vi "Autonomous Independent.vi"   [LabVIEW 2017] (continued)
                tunnel: [w1142] -> w956
                tunnel: [w1141] -> w955
                tunnel: w958 -> [w1156]
                tunnel: w957 -> [w1155]
                tunnel: [w1154] -> w954
                tunnel: [w1153] -> w953
                tunnel: [w1152] -> w952
                tunnel: w956 -> [w1152]
                tunnel: [w1151] -> w951
                tunnel: w955 -> [w1151]
                tunnel: w954 -> [w1164]
                tunnel: w953 -> [w1163]
                tunnel: [w1162] -> w950
                tunnel: w952 -> [w1162]
                tunnel: [w1161] -> w949
                tunnel: w951 -> [w1161]
                tunnel: [w1160] -> w948
                tunnel: [w1159] -> w947
                tunnel: w950 -> [w1184]
                tunnel: w949 -> [w1183]
                tunnel: [w1182] -> w946
                tunnel: w948 -> [w1182]
                tunnel: [w1181] -> w945
                tunnel: w947 -> [w1181]
                tunnel: [w1180] -> w944
                tunnel: [w1179] -> w943
                tunnel: w946 -> [w1192]
                tunnel: w945 -> [w1191]
                tunnel: w944 -> [w1190]
                tunnel: w943 -> [w1189]
                tunnel: [w1188] -> w942
                tunnel: [w1187] -> w941
                tunnel: [w1186] -> w940
                tunnel: [w1185] -> w939
                tunnel: [w1198] -> w935
                tunnel: w942 -> [w1198]
                tunnel: [w1197] -> w936
                tunnel: w941 -> [w1197]
                tunnel: [w1196] -> w937
                tunnel: w940 -> [w1196]
                tunnel: [w1195] -> w938
                tunnel: w939 -> [w1195]
                tunnel: [w1206] -> w934
                tunnel: [w1202] -> w933
                tunnel: [w1201] -> w932
                tunnel: [w1205] -> w931
                tunnel: w938 -> [w1201]
                tunnel: w937 -> [w1202]
                tunnel: w936 -> [w1203]
                tunnel: w935 -> [w1204]
                tunnel: w934 -> [w1214]
                tunnel: w933 -> [w1213]
                tunnel: w932 -> [w1212]
                tunnel: [w1211] -> w930
                tunnel: w931 -> [w1211]
                tunnel: [w1210] -> w929
                tunnel: [w1209] -> w928
                tunnel: [w1208] -> w927
                tunnel: w930 -> [w1224]
                tunnel: w929 -> [w1223]
                tunnel: w928 -> [w1222]
                tunnel: w927 -> [w1221]
                tunnel: [w1220] -> w926
                tunnel: [w1219] -> w925
                tunnel: [w1218] -> w924
                tunnel: [w1217] -> w923
                tunnel: w926 -> [w1233]
                tunnel: w925 -> [w1232]
                tunnel: [w1231] -> w922
                tunnel: w924 -> [w1231]
                tunnel: [w1230] -> w921
                tunnel: w923 -> [w1230]
                tunnel: [w1229] -> w920
                tunnel: [w1228] -> w919
                tunnel: w922 -> [w1246]
                tunnel: w921 -> [w1245]
                tunnel: [w1244] -> w918
                tunnel: w920 -> [w1244]
                tunnel: [w1243] -> w917
                tunnel: w919 -> [w1243]
                tunnel: [w1242] -> w916
                tunnel: [w1241] -> w915
                tunnel: w918 -> [w1260]
                tunnel: w917 -> [w1259]
                tunnel: w916 -> [w1258]
                tunnel: w915 -> [w1257]
                tunnel: [w1256] -> w914
                tunnel: [w1255] -> w913
                tunnel: [w1254] -> w912
                tunnel: [w1253] -> w911
                tunnel: [w1266] -> w910
                tunnel: w914 -> [w1267]
                tunnel: [w1265] -> w909
                tunnel: w913 -> [w1265]
                tunnel: [w1264] -> w908
                tunnel: w912 -> [w1264]
                tunnel: [w1263] -> w907
                tunnel: w911 -> [w1263]
                tunnel: [w1278] -> w906
                tunnel: w910 -> [w1278]
                tunnel: [w1277] -> w905
                tunnel: w909 -> [w1277]
                tunnel: [w1276] -> w904
                tunnel: w908 -> [w1276]
                tunnel: [w1275] -> w903
                tunnel: w907 -> [w1275]
                tunnel: w906 -> [w1284]
                tunnel: w905 -> [w1283]
                tunnel: w904 -> [w1282]
                tunnel: w903 -> [w1281]
                frame #0 {
                  n287 = call "PID Distance.vi"("Distance"=20.0, "Angle"=0.0, "RightEncoder"=w1015, "LeftEncoder"=w1016, "GyroDevRef"=w1018, "RobotDriveDevRef"=w1017) -> ("RightEncoder 2"=w1011:T11, "LeftEncoder 2"=w1012:T11, "GyroDevRef 2"=w1013:T8, "RobotDriveDevRef 2"=w1014:T1)  [unwired: 2 in]
                }
                frame #1 {
                  w1027 = 0.0 ("Left axis value")
                  n288 = global write "Robot Global Data.vi" "Raise_Mast"(TRUE ("Current State")) -> ()
                  n289 = Wait (ms)(milliseconds to wait=u32 100) -> ()  [unwired: 1 out]
                  n290 = call <vilib>:"WPI_RobotDriveTankDrive.vi"("Right axis value"=w1027, "Left axis value"=w1027, "RobotDriveDevRef"=w1025) -> ("RobotDriveDevRef"=w1026:T1)  [unwired: 6 in, 2 out]
                }
                frame #2 {
                  n291 = call "PID turning.vi"("Angle"=-50.0, "GyroDevRef"=w1032, "RobotDriveDevRef"=w1031) -> ("GyroDevRef 2"=w1029:T8, "RobotDriveDevRef 2"=w1030:T1)  [unwired: 7 in]
                  n292 = global write "Robot Global Data.vi" "Raise_Mast"(TRUE ("Current State")) -> ()
                }
                frame #3 {
                  w1038 = 0.0 ("Left axis value")
                  n293 = call <vilib>:"WPI_EncoderReset.vi"("EncoderDevRef"=w1043) -> ("EncoderDevRef"=w1040:T11)  [unwired: 9 in, 1 out]
                  n294 = call <vilib>:"WPI_EncoderReset.vi"("EncoderDevRef"=w1042) -> ("EncoderDevRef"=w1041:T11)  [unwired: 9 in, 1 out]
                  n295 = Wait (ms)(milliseconds to wait=u32 10) -> ()  [unwired: 1 out]
                  n296 = call <vilib>:"WPI_RobotDriveTankDrive.vi"("Right axis value"=w1038, "Left axis value"=w1038, "RobotDriveDevRef"=w1044) -> ("RobotDriveDevRef"=w1039:T1)  [unwired: 6 in, 2 out]
                }
                frame #4 {
                  n297 = call "PID Distance.vi"("Distance"=75.0, "Angle"=-50.0, "RightEncoder"=w1051, "LeftEncoder"=w1050, "GyroDevRef"=w1053, "RobotDriveDevRef"=w1052) -> ("RightEncoder 2"=w1046:T11, "LeftEncoder 2"=w1047:T11, "GyroDevRef 2"=w1049:T8, "RobotDriveDevRef 2"=w1048:T1)  [unwired: 2 in]
                  n298 = global write "Robot Global Data.vi" "Raise_Mast"(TRUE ("Current State")) -> ()
                }
                frame #5 {
                  n299 = global read "Robot Global Data.vi" "Axes"() -> (w1063:dbl[])
                  n300 = global write "Robot Global Data.vi" "Raise_Mast"(TRUE ("Current State")) -> ()
                  n301 = Array To Cluster(array=w1063) -> (cluster=w1064:T15)
                  n302 = Bundle By Name(cluster=w1064, "Axes[1]"=-1.0) -> (w1061:T15)
                  n303 = Cluster To Array(cluster=w1061) -> (array=w1062:dbl[])
                  n304 = call "PID turning.vi"("Angle"=0.0, "GyroDevRef"=w1065, "RobotDriveDevRef"=w1066) -> ("GyroDevRef 2"=w1057:T8, "RobotDriveDevRef 2"=w1058:T1)  [unwired: 7 in]
                  n305 = global write "Robot Global Data.vi" "Axes"(w1062) -> ()
                }
                frame #6 {
                  n306 = global read "Robot Global Data.vi" "Axes"() -> (w1073:dbl[])
                  n307 = global write "Robot Global Data.vi" "Lift_Position"(2.0) -> ()
                  n308 = Array To Cluster(array=w1073) -> (cluster=w1072:T15)
                  n309 = Bundle By Name(cluster=w1072, "Axes[1]"=-1.0) -> (w1075:T15)
                  n310 = Cluster To Array(cluster=w1075) -> (array=w1074:dbl[])
                  n311 = call <vilib>:"WPI_EncoderReset.vi"("EncoderDevRef"=w1070) -> ("EncoderDevRef"=w1080:T11)  [unwired: 9 in, 1 out]
                  n312 = global write "Robot Global Data.vi" "Axes"(w1074) -> ()
                  n313 = call <vilib>:"WPI_EncoderReset.vi"("EncoderDevRef"=w1071) -> ("EncoderDevRef"=w1081:T11)  [unwired: 9 in, 1 out]
                }
                frame #7 {
                  n314 = call "PID Distance.vi"("Distance"=50.0, "Angle"=0.0, "RightEncoder"=w1085, "LeftEncoder"=w1086, "GyroDevRef"=w1088, "RobotDriveDevRef"=w1087) -> ("RightEncoder 2"=w1082:T11, "LeftEncoder 2"=w1083:T11, "GyroDevRef 2"=w1084:T8, "RobotDriveDevRef 2"=w1089:T1)  [unwired: 2 in]
                }
                frame #8 {
                  w1104 = 0.0 ("Left axis value")
                  n315 = global read "Robot Global Data.vi" "Axes"() -> (w1100:dbl[])
                  n316 = global write "Robot Global Data.vi" "Lift_Position"(2.0) -> ()
                  n317 = Wait (ms)(milliseconds to wait=u32 250) -> ()  [unwired: 1 out]
                  n318 = Array To Cluster(array=w1100) -> (cluster=w1099:T15)
                  n319 = Bundle By Name(cluster=w1099, "Axes[1]"=1.0) -> (w1097:T15)
                  n320 = Cluster To Array(cluster=w1097) -> (array=w1096:dbl[])
                  n321 = call <vilib>:"WPI_RobotDriveTankDrive.vi"("Right axis value"=w1104, "Left axis value"=w1104, "RobotDriveDevRef"=w1103) -> ("RobotDriveDevRef"=w1095:T1)  [unwired: 6 in, 2 out]
                  n322 = global write "Robot Global Data.vi" "Axes"(w1096) -> ()
                }
                frame #9 {
                  n323 = global write "Robot Global Data.vi" "Current State"(FALSE ("Current State")) -> ()
                  n324 = Wait (ms)(milliseconds to wait=u32 500) -> ()  [unwired: 1 out]
                }
                frame #10 {
                  n325 = global read "Robot Global Data.vi" "Axes"() -> (w1126:dbl[])
                  n326 = global write "Robot Global Data.vi" "Lift_Position"(1.0) -> ()
                  n327 = Array To Cluster(array=w1126) -> (cluster=w1125:T15)
                  n328 = Bundle By Name(cluster=w1125, "Axes[1]"=0.0) -> (w1123:T15)
                  n329 = Cluster To Array(cluster=w1123) -> (array=w1122:dbl[])
                  n330 = call "PID Distance.vi"("Distance"=0.0, "Angle"=0.0, "RightEncoder"=w1118, "LeftEncoder"=w1117, "GyroDevRef"=w1116, "RobotDriveDevRef"=w1115) -> ("RightEncoder 2"=w1111:T11, "LeftEncoder 2"=w1112:T11, "GyroDevRef 2"=w1113:T8, "RobotDriveDevRef 2"=w1114:T1)  [unwired: 2 in]
                  n331 = global write "Robot Global Data.vi" "Axes"(w1122) -> ()
                }
                frame #11 {
                  n332 = call "PID turning.vi"("Angle"=-50.0, "GyroDevRef"=w1131, "RobotDriveDevRef"=w1132) -> ("GyroDevRef 2"=w1127:T8, "RobotDriveDevRef 2"=w1128:T1)  [unwired: 7 in]
                }
                frame #12 {
                  n333 = call <vilib>:"WPI_EncoderReset.vi"("EncoderDevRef"=w1139) -> ("EncoderDevRef"=w1135:T11)  [unwired: 9 in, 1 out]
                  n334 = call <vilib>:"WPI_EncoderReset.vi"("EncoderDevRef"=w1138) -> ("EncoderDevRef"=w1134:T11)  [unwired: 9 in, 1 out]
                }
                frame #13 {
                  n335 = global write "Robot Global Data.vi" "Lift_Position"(0.0) -> ()
                  n336 = call "PID Distance.vi"("Distance"=-75.0, "Angle"=-50.0, "RightEncoder"=w1145, "LeftEncoder"=w1146, "GyroDevRef"=w1147, "RobotDriveDevRef"=w1148) -> ("RightEncoder 2"=w1141:T11, "LeftEncoder 2"=w1142:T11, "GyroDevRef 2"=w1143:T8, "RobotDriveDevRef 2"=w1144:T1)  [unwired: 2 in]
                }
                frame #14 {
                  n337 = call "PID turning.vi"("Angle"=0.0, "GyroDevRef"=w1155, "RobotDriveDevRef"=w1156) -> ("GyroDevRef 2"=w1153:T8, "RobotDriveDevRef 2"=w1154:T1)  [unwired: 7 in]
                }
                frame #15 {
                  n338 = global read "Robot Global Data.vi" "PIXY Output"() -> (w1165:T16)
                  n339 = Unbundle By Name(w1165) -> ("SIGNATURE NUMBER"=w1167:u16)
                  n340 = global read "Robot Global Data.vi" "Cube Signature"() -> (w1158:dbl)
                  n341 = Equal?(x=w1167, y=w1158) -> (x = y?=w1166:bool)
                  n342 = case shown="True" w1166 {
                    tunnel: [w1174 w1177] -> w1159
                    tunnel: [w1175 w1176] -> w1160
                    tunnel: w1164 -> [w1169 w1176]
                    tunnel: w1163 -> [w1168 w1177]
                    frame True {
                      n343 = call <vilib>:"WPI_GyroGetAngle.vi"("GyroDevRef"=w1168) -> ("Angle"=w1173:dbl, "GyroDevRef"=w1174:T8)  [unwired: 6 in, 3 out]
                      n344 = In Range and Coerce(upper limit=-1.0, x=w1173, lower limit=-5.0) -> (coerced(x)=w1172:dbl)  [unwired: 1 out]
                      n345 = global write "Robot Global Data.vi" "Tracked Angle"(w1172) -> ()
                      n346 = call "PID vision.vi"("RobotDriveDevRef in"=w1169) -> ("RobotDriveDevRef out"=w1175:T1)  [unwired: 9 in, 1 out]
                    }
                    frame False {
                      n347 = global write "Robot Global Data.vi" "Tracked Angle"(-2.0) -> ()
                    }
                  }
                }
                frame #16 {
                  n348 = call <vilib>:"WPI_EncoderReset.vi"("EncoderDevRef"=w1184) -> ("EncoderDevRef"=w1180:T11)  [unwired: 9 in, 1 out]
                  n349 = call <vilib>:"WPI_EncoderReset.vi"("EncoderDevRef"=w1183) -> ("EncoderDevRef"=w1179:T11)  [unwired: 9 in, 1 out]
                }
                frame #17 {
                  n350 = global read "Robot Global Data.vi" "Tracked Angle"() -> (w1193:dbl)
                  n351 = call "PID Distance.vi"("Distance"=52.0, "Angle"=w1193, "RightEncoder"=w1189, "LeftEncoder"=w1190, "GyroDevRef"=w1191, "RobotDriveDevRef"=w1192) -> ("RightEncoder 2"=w1185:T11, "LeftEncoder 2"=w1186:T11, "GyroDevRef 2"=w1187:T8, "RobotDriveDevRef 2"=w1188:T1)  [unwired: 2 in]
                }
                frame #18 {
                  n352 = global write "Robot Global Data.vi" "Current State"(TRUE ("Current State")) -> ()
                  n353 = Wait (ms)(milliseconds to wait=u32 750) -> ()  [unwired: 1 out]
                }
                frame #19 {
                  n354 = call "PID turning.vi"("Angle"=-90.0, "GyroDevRef"=w1203, "RobotDriveDevRef"=w1204) -> ("GyroDevRef 2"=w1205:T8, "RobotDriveDevRef 2"=w1206:T1)  [unwired: 7 in]
                }
                frame #20 {
                  w1215 = 0.0 ("Left axis value")
                  n355 = call <vilib>:"WPI_EncoderReset.vi"("EncoderDevRef"=w1213) -> ("EncoderDevRef"=w1209:T11)  [unwired: 9 in, 1 out]
                  n356 = call <vilib>:"WPI_RobotDriveTankDrive.vi"("Right axis value"=w1215, "Left axis value"=w1215, "RobotDriveDevRef"=w1214) -> ("RobotDriveDevRef"=w1210:T1)  [unwired: 6 in, 2 out]
                  n357 = Wait (ms)(milliseconds to wait=u32 10) -> ()  [unwired: 1 out]
                  n358 = call <vilib>:"WPI_EncoderReset.vi"("EncoderDevRef"=w1212) -> ("EncoderDevRef"=w1208:T11)  [unwired: 9 in, 1 out]
                }
                frame #21 {
                  n359 = call "PID Distance.vi"("Distance"=50.0, "Angle"=-90.0, "RightEncoder"=w1221, "LeftEncoder"=w1222, "GyroDevRef"=w1224, "RobotDriveDevRef"=w1223) -> ("RightEncoder 2"=w1217:T11, "LeftEncoder 2"=w1218:T11, "GyroDevRef 2"=w1219:T8, "RobotDriveDevRef 2"=w1220:T1)  [unwired: 2 in]
                  n360 = global write "Robot Global Data.vi" "Raise_Mast"(TRUE ("Current State")) -> ()
                }
                frame #22 {
                  n361 = global read "Robot Global Data.vi" "Axes"() -> (w1238:dbl[])
                  n362 = global write "Robot Global Data.vi" "Raise_Mast"(TRUE ("Current State")) -> ()
                  n363 = Array To Cluster(array=w1238) -> (cluster=w1239:T15)
                  n364 = Bundle By Name(cluster=w1239, "Axes[1]"=-1.0) -> (w1236:T15)
                  n365 = Cluster To Array(cluster=w1236) -> (array=w1237:dbl[])
                  n366 = call "PID turning.vi"("Angle"=0.0, "GyroDevRef"=w1232, "RobotDriveDevRef"=w1233) -> ("GyroDevRef 2"=w1228:T8, "RobotDriveDevRef 2"=w1229:T1)  [unwired: 7 in]
                  n367 = global write "Robot Global Data.vi" "Axes"(w1237) -> ()
                }
                frame #23 {
                  n368 = global read "Robot Global Data.vi" "Axes"() -> (w1248:dbl[])
                  n369 = global write "Robot Global Data.vi" "Lift_Position"(2.0) -> ()
                  n370 = Array To Cluster(array=w1248) -> (cluster=w1247:T15)
                  n371 = Bundle By Name(cluster=w1247, "Axes[1]"=-1.0) -> (w1250:T15)
                  n372 = Cluster To Array(cluster=w1250) -> (array=w1249:dbl[])
                  n373 = call <vilib>:"WPI_EncoderReset.vi"("EncoderDevRef"=w1245) -> ("EncoderDevRef"=w1241:T11)  [unwired: 9 in, 1 out]
                  n374 = global write "Robot Global Data.vi" "Axes"(w1249) -> ()
                  n375 = call <vilib>:"WPI_EncoderReset.vi"("EncoderDevRef"=w1246) -> ("EncoderDevRef"=w1242:T11)  [unwired: 9 in, 1 out]
                }
                frame #24 {
                  n376 = call "PID Distance.vi"("Distance"=40.0, "Angle"=0.0, "RightEncoder"=w1257, "LeftEncoder"=w1258, "GyroDevRef"=w1259, "RobotDriveDevRef"=w1260) -> ("RightEncoder 2"=w1253:T11, "LeftEncoder 2"=w1254:T11, "GyroDevRef 2"=w1255:T8, "RobotDriveDevRef 2"=w1256:T1)  [unwired: 2 in]
                }
                frame #25 {
                  w1274 = 0.0 ("Left axis value")
                  n377 = global read "Robot Global Data.vi" "Axes"() -> (w1272:dbl[])
                  n378 = global write "Robot Global Data.vi" "Lift_Position"(2.0) -> ()
                  n379 = Array To Cluster(array=w1272) -> (cluster=w1271:T15)
                  n380 = Bundle By Name(cluster=w1271, "Axes[1]"=1.0) -> (w1269:T15)
                  n381 = Cluster To Array(cluster=w1269) -> (array=w1268:dbl[])
                  n382 = call <vilib>:"WPI_RobotDriveTankDrive.vi"("Right axis value"=w1274, "Left axis value"=w1274, "RobotDriveDevRef"=w1267) -> ("RobotDriveDevRef"=w1266:T1)  [unwired: 6 in, 2 out]
                  n383 = global write "Robot Global Data.vi" "Axes"(w1268) -> ()
                }
                frame #26 {
                  n384 = global write "Robot Global Data.vi" "Current State"(FALSE ("Current State")) -> ()
                  n385 = Wait (ms)(milliseconds to wait=u32 500) -> ()  [unwired: 1 out]
                }
                frame #27 {
                  n386 = global read "Robot Global Data.vi" "Axes"() -> (w1292:dbl[])
                  n387 = call "PID Distance.vi"("Distance"=0.0, "Angle"=0.0, "RightEncoder"=w1281, "LeftEncoder"=w1282, "GyroDevRef"=w1283, "RobotDriveDevRef"=w1284) -> ()  [unwired: 2 in, 4 out]
                  n388 = global write "Robot Global Data.vi" "Lift_Position"(0.0) -> ()
                  n389 = Array To Cluster(array=w1292) -> (cluster=w1291:T15)
                  n390 = Bundle By Name(cluster=w1291, "Axes[1]"=0.0) -> (w1286:T15)
                  n391 = Cluster To Array(cluster=w1286) -> (array=w1285:dbl[])
                  n392 = global write "Robot Global Data.vi" "Axes"(w1285) -> ()
                }
              }
            }
          }
        }
      }
    }
    frame "Left Scale C" {
      n393 = flat-sequence {
        tunnel: w1299 -> [w1328]
        tunnel: w1296 -> [w1326]
        tunnel: w1297 -> [w1325]
        tunnel: w1298 -> [w1324]
        tunnel: [w1323] -> w1303
        tunnel: [w1322] -> w1302
        tunnel: [w1321] -> w1301
        tunnel: [w1320] -> w1300
        tunnel: w1295 -> [w1313]
        tunnel: w1294 -> [w1330]
        tunnel: w1303 -> [w1334]
        tunnel: w1302 -> [w1333]
        tunnel: w1301 -> [w1332]
        tunnel: w1300 -> [w1331]
        tunnel: w1293 -> [w1329]
        frame #0 {
          w1327 = 0.0 ("Left axis value")
          n394 = global read "Robot Global Data.vi" "Axes"() -> (w1306:dbl[])
          n395 = Multiply(x=w1313, y=1000.0) -> (x*y=w1314:dbl)
          n396 = global write "Robot Global Data.vi" "Lift_Position"(0.0) -> ()
          n397 = global write "Robot Global Data.vi" "Current State"(TRUE ("Current State")) -> ()
          n398 = global write "Robot Global Data.vi" "Raise_Mast"(FALSE ("Current State")) -> ()
          n399 = Wait (ms)(milliseconds to wait=u32 100) -> ()  [unwired: 1 out]
          n400 = Array To Cluster(array=w1306) -> (cluster=w1305:T15)
          n401 = Bundle By Name(cluster=w1305, "Axes[1]"=-1.0) -> (w1308:T15)
          n402 = Greater?(x=w1314, y=11000.0) -> (0:w1316:bool)
          n403 = Equal?(x=w1314, y=0.0) -> (x = y?=w1317:bool)
          n404 = Or(x=w1316, y=w1317) -> ()  [unwired: 1 out]
          n405 = Cluster To Array(cluster=w1308) -> (array=w1307:dbl[])
          n406 = call <vilib>:"WPI_GyroReset.vi"("GyroDevRef"=w1324) -> ("GyroDevRef"=w1320:T8)  [unwired: 9 in, 1 out]
          n407 = call <vilib>:"WPI_EncoderReset.vi"("EncoderDevRef"=w1326) -> ("EncoderDevRef"=w1322:T11)  [unwired: 9 in, 1 out]
          n408 = global write "Robot Global Data.vi" "Axes"(w1307) -> ()
          n409 = call <vilib>:"WPI_EncoderReset.vi"("EncoderDevRef"=w1325) -> ("EncoderDevRef"=w1321:T11)  [unwired: 9 in, 1 out]
          n410 = call <vilib>:"WPI_RobotDriveTankDrive.vi"("Right axis value"=w1327, "Left axis value"=w1327, "RobotDriveDevRef"=w1328) -> ("RobotDriveDevRef"=w1323:T1)  [unwired: 6 in, 2 out]
        }
        frame #1 {
          n411 = case shown="\"R\"" w1330 {
            tunnel: w1334 -> [w1339 w1407 w1546]
            tunnel: w1333 -> [w1336 w1404 w1548]
            tunnel: w1332 -> [w1337 w1405 w1547]
            tunnel: w1331 -> [w1338 w1406 w1545]
            tunnel: w1329 -> [w1335 _ _]
            frame "R" {
              n412 = flat-sequence {
                tunnel: w1336 -> [w1361]
                tunnel: w1337 -> [w1362]
                tunnel: w1338 -> [w1363]
                tunnel: w1339 -> [w1364]
                tunnel: [w1357] -> w1355
                tunnel: [w1358] -> w1354
                tunnel: [w1359] -> w1353
                tunnel: [w1360] -> w1352
                tunnel: [w1374] -> w1351
                tunnel: [w1373] -> w1350
                tunnel: [w1371] -> w1349
                tunnel: [w1372] -> w1348
                tunnel: w1355 -> [w1370]
                tunnel: w1354 -> [w1369]
                tunnel: w1353 -> [w1368]
                tunnel: w1352 -> [w1367]
                tunnel: w1351 -> [w1380]
                tunnel: w1350 -> [w1381]
                tunnel: [w1384] -> w1347
                tunnel: w1349 -> [w1384]
                tunnel: [w1383] -> w1346
                tunnel: w1348 -> [w1383]
                tunnel: [w1378] -> w1345
                tunnel: [w1379] -> w1344
                tunnel: w1347 -> [w1391]
                tunnel: w1346 -> [w1390]
                tunnel: [w1389] -> w1343
                tunnel: [w1388] -> w1342
                tunnel: [w1387] -> w1341
                tunnel: w1345 -> [w1387]
                tunnel: [w1385] -> w1340
                tunnel: w1344 -> [w1385]
                tunnel: w1335 -> [_]
                tunnel: w1340 -> [w1395]
                tunnel: w1341 -> [w1394]
                tunnel: w1342 -> [w1393]
                tunnel: w1343 -> [w1392]
                frame #0 {
                  n413 = global write "Robot Global Data.vi" "Raise_Mast"(FALSE ("Current State")) -> ()
                  n414 = call "PID Distance.vi"("Distance"=20.0, "Angle"=0.0, "RightEncoder"=w1361, "LeftEncoder"=w1362, "GyroDevRef"=w1363, "RobotDriveDevRef"=w1364) -> ("RightEncoder 2"=w1360:T11, "LeftEncoder 2"=w1359:T11, "GyroDevRef 2"=w1358:T8, "RobotDriveDevRef 2"=w1357:T1)  [unwired: 2 in]
                }
                frame #1 {
                  n415 = global write "Robot Global Data.vi" "Raise_Mast"(TRUE ("Current State")) -> ()
                  n416 = call "PID Distance.vi"("Distance"=225.0, "Angle"=0.0, "RightEncoder"=w1367, "LeftEncoder"=w1368, "GyroDevRef"=w1369, "RobotDriveDevRef"=w1370) -> ("RightEncoder 2"=w1371:T11, "LeftEncoder 2"=w1372:T11, "GyroDevRef 2"=w1373:T8, "RobotDriveDevRef 2"=w1374:T1)  [unwired: 2 in]
                }
                frame #2 {
                  n417 = call "PID turning.vi"("Angle"=90.0, "GyroDevRef"=w1381, "RobotDriveDevRef"=w1380) -> ("GyroDevRef 2"=w1378:T8, "RobotDriveDevRef 2"=w1379:T1)  [unwired: 7 in]
                }
                frame #3 {
                  n418 = call <vilib>:"WPI_EncoderReset.vi"("EncoderDevRef"=w1390) -> ("EncoderDevRef"=w1388:T11)  [unwired: 9 in, 1 out]
                  n419 = Wait (ms)(milliseconds to wait=u32 10) -> ()  [unwired: 1 out]
                  n420 = call <vilib>:"WPI_EncoderReset.vi"("EncoderDevRef"=w1391) -> ("EncoderDevRef"=w1389:T11)  [unwired: 9 in, 1 out]
                }
                frame #4 {
                  n421 = global read "Robot Global Data.vi" "Axes"() -> (w1399:dbl[])
                  n422 = global write "Robot Global Data.vi" "Lift_Position"(2.0) -> ()
                  n423 = call "PID Distance.vi"("Distance"=100.0, "Angle"=90.0, "RightEncoder"=w1392, "LeftEncoder"=w1393, "GyroDevRef"=w1394, "RobotDriveDevRef"=w1395) -> ()  [unwired: 2 in, 4 out]
                  n424 = Array To Cluster(array=w1399) -> (cluster=w1398:T15)
                  n425 = Bundle By Name(cluster=w1398, "Axes[1]"=-1.0) -> (w1397:T15)
                  n426 = Cluster To Array(cluster=w1397) -> (array=w1396:dbl[])
                  n427 = global write "Robot Global Data.vi" "Axes"(w1396) -> ()
                }
              }
            }
            frame "L" {
              n428 = flat-sequence {
                tunnel: [w1455] -> w1447
                tunnel: [w1452] -> w1446
                tunnel: [w1453] -> w1445
                tunnel: [w1454] -> w1444
                tunnel: w1407 -> [w1451]
                tunnel: w1406 -> [w1450]
                tunnel: w1405 -> [w1449]
                tunnel: w1404 -> [w1448]
                tunnel: [w1462] -> w1443
                tunnel: [w1459] -> w1442
                tunnel: [w1460] -> w1441
                tunnel: [w1461] -> w1440
                tunnel: w1447 -> [w1466]
                tunnel: w1446 -> [w1463]
                tunnel: w1445 -> [w1464]
                tunnel: w1444 -> [w1465]
                tunnel: [w1473] -> w1436
                tunnel: [w1472] -> w1437
                tunnel: [w1470] -> w1438
                tunnel: [w1471] -> w1439
                tunnel: w1443 -> [w1477]
                tunnel: w1442 -> [w1474]
                tunnel: w1441 -> [w1475]
                tunnel: w1440 -> [w1476]
                tunnel: [w1485] -> w1435
                tunnel: w1439 -> [w1481]
                tunnel: w1438 -> [w1482]
                tunnel: w1437 -> [w1484]
                tunnel: w1436 -> [w1486]
                tunnel: [w1483] -> w1434
                tunnel: [w1482] -> w1433
                tunnel: [w1481] -> w1432
                tunnel: w1435 -> [w1496]
                tunnel: [w1496] -> w1431
                tunnel: w1434 -> [w1495]
                tunnel: [w1495] -> w1430
                tunnel: [w1494] -> w1429
                tunnel: [w1493] -> w1428
                tunnel: w1433 -> [w1491]
                tunnel: w1432 -> [w1490]
                tunnel: w1431 -> [w1502]
                tunnel: [w1500] -> w1427
                tunnel: w1430 -> [w1501]
                tunnel: [w1499] -> w1426
                tunnel: w1429 -> [w1504]
                tunnel: w1428 -> [w1503]
                tunnel: [w1498] -> w1425
                tunnel: [w1497] -> w1424
                tunnel: w1427 -> [w1511]
                tunnel: [w1510] -> w1423
                tunnel: [w1509] -> w1422
                tunnel: w1426 -> [w1509]
                tunnel: [w1508] -> w1421
                tunnel: w1425 -> [w1508]
                tunnel: [w1507] -> w1420
                tunnel: w1424 -> [w1507]
                tunnel: [w1522] -> w1419
                tunnel: w1423 -> [w1522]
                tunnel: [w1521] -> w1418
                tunnel: w1422 -> [w1521]
                tunnel: [w1520] -> w1417
                tunnel: w1421 -> [w1520]
                tunnel: [w1519] -> w1416
                tunnel: w1420 -> [w1519]
                tunnel: w1419 -> [w1527]
                tunnel: w1418 -> [w1528]
                tunnel: [w1528] -> w1415
                tunnel: [w1527] -> w1414
                tunnel: [w1526] -> w1413
                tunnel: w1417 -> [w1526]
                tunnel: [w1525] -> w1412
                tunnel: w1416 -> [w1525]
                tunnel: [w1541] -> w1411
                tunnel: w1415 -> [w1543]
                tunnel: w1414 -> [w1542]
                tunnel: w1413 -> [w1538]
                tunnel: w1412 -> [w1537]
                tunnel: [w1536] -> w1410
                tunnel: [w1535] -> w1409
                tunnel: [w1534] -> w1408
                tunnel: w1408 -> [_]
                tunnel: w1409 -> [_]
                tunnel: w1410 -> [_]
                tunnel: w1411 -> [_]
                frame #0 {
                  n429 = call "PID Distance.vi"("Distance"=20.0, "Angle"=-2.0, "RightEncoder"=w1448, "LeftEncoder"=w1449, "GyroDevRef"=w1450, "RobotDriveDevRef"=w1451) -> ("RightEncoder 2"=w1452:T11, "LeftEncoder 2"=w1453:T11, "GyroDevRef 2"=w1454:T8, "RobotDriveDevRef 2"=w1455:T1)  [unwired: 2 in]
                }
                frame #1 {
                  n430 = call "PID Distance.vi"("Distance"=100.0, "Angle"=-2.0, "RightEncoder"=w1463, "LeftEncoder"=w1464, "GyroDevRef"=w1465, "RobotDriveDevRef"=w1466) -> ("RightEncoder 2"=w1459:T11, "LeftEncoder 2"=w1460:T11, "GyroDevRef 2"=w1461:T8, "RobotDriveDevRef 2"=w1462:T1)  [unwired: 2 in]
                  n431 = global write "Robot Global Data.vi" "Raise_Mast"(TRUE ("Current State")) -> ()
                }
                frame #2 {
                  n432 = global write "Robot Global Data.vi" "Lift_Position"(2.0) -> ()
                  n433 = call "PID Distance.vi"("Distance"=300.0, "Angle"=-2.0, "RightEncoder"=w1474, "LeftEncoder"=w1475, "GyroDevRef"=w1476, "RobotDriveDevRef"=w1477) -> ("RightEncoder 2"=w1470:T11, "LeftEncoder 2"=w1471:T11, "GyroDevRef 2"=w1472:T8, "RobotDriveDevRef 2"=w1473:T1)  [unwired: 2 in]
                  n434 = global write "Robot Global Data.vi" "Raise_Mast"(TRUE ("Current State")) -> ()
                }
                frame #3 {
                  n435 = call "PID turning.vi"("Angle"=90.0, "GyroDevRef"=w1484, "RobotDriveDevRef"=w1486) -> ("GyroDevRef 2"=w1483:T8, "RobotDriveDevRef 2"=w1485:T1)  [unwired: 7 in]
                  n436 = global write "Robot Global Data.vi" "Lift_Position"(3.0) -> ()
                  n437 = global write "Robot Global Data.vi" "Raise_Mast"(TRUE ("Current State")) -> ()
                }
                frame #4 {
                  n438 = call <vilib>:"WPI_EncoderReset.vi"("EncoderDevRef"=w1490) -> ("EncoderDevRef"=w1493:T11)  [unwired: 9 in, 1 out]
                  n439 = Wait (ms)(milliseconds to wait=u32 100) -> ()  [unwired: 1 out]
                  n440 = call <vilib>:"WPI_EncoderReset.vi"("EncoderDevRef"=w1491) -> ("EncoderDevRef"=w1494:T11)  [unwired: 9 in, 1 out]
                }
                frame #5 {
                  n441 = call "PID Distance.vi"("Distance"=25.0, "Angle"=90.0, "RightEncoder"=w1504, "LeftEncoder"=w1503, "GyroDevRef"=w1501, "RobotDriveDevRef"=w1502) -> ("RightEncoder 2"=w1497:T11, "LeftEncoder 2"=w1498:T11, "GyroDevRef 2"=w1499:T8, "RobotDriveDevRef 2"=w1500:T1)  [unwired: 2 in]
                }
                frame #6 {
                  w1512 = 0.0 ("Left axis value")
                  n442 = global read "Robot Global Data.vi" "Axes"() -> (w1515:dbl[])
                  n443 = Wait (ms)(milliseconds to wait=u32 500) -> ()  [unwired: 1 out]
                  n444 = Array To Cluster(array=w1515) -> (cluster=w1514:T15)
                  n445 = Bundle By Name(cluster=w1514, "Axes[1]"=0.25) -> (w1517:T15)
                  n446 = Cluster To Array(cluster=w1517) -> (array=w1516:dbl[])
                  n447 = call <vilib>:"WPI_RobotDriveTankDrive.vi"("Right axis value"=w1512, "Left axis value"=w1512, "RobotDriveDevRef"=w1511) -> ("RobotDriveDevRef"=w1510:T1)  [unwired: 6 in, 2 out]
                  n448 = global write "Robot Global Data.vi" "Axes"(w1516) -> ()
                }
                frame #7 {
                  n449 = global write "Robot Global Data.vi" "Current State"(FALSE ("Current State")) -> ()
                  n450 = Wait (ms)(milliseconds to wait=u32 400) -> ()  [unwired: 1 out]
                }
                frame #8 {
                  n451 = global read "Robot Global Data.vi" "Axes"() -> (w1530:dbl[])
                  n452 = Array To Cluster(array=w1530) -> (cluster=w1529:T15)
                  n453 = Bundle By Name(cluster=w1529, "Axes[1]"=-1.0) -> (w1532:T15)
                  n454 = Cluster To Array(cluster=w1532) -> (array=w1531:dbl[])
                  n455 = global write "Robot Global Data.vi" "Axes"(w1531) -> ()
                }
                frame #9 {
                  n456 = call "PID Distance.vi"("Distance"=0.0, "Angle"=90.0, "RightEncoder"=w1537, "LeftEncoder"=w1538, "GyroDevRef"=w1543, "RobotDriveDevRef"=w1542) -> ("RightEncoder 2"=w1534:T11, "LeftEncoder 2"=w1535:T11, "GyroDevRef 2"=w1536:T8, "RobotDriveDevRef 2"=w1541:T1)  [unwired: 2 in]
                }
                frame #10 {
                  n457 = global write "Robot Global Data.vi" "Lift_Position"(1.0) -> ()
                }
              }
            }
            frame Default {
              n458 = flat-sequence {
                tunnel: w1546 -> [w1554]
                tunnel: w1545 -> [w1553]
                tunnel: w1547 -> [w1551]
                tunnel: [w1552] -> w1549
                tunnel: w1548 -> [w1550]
                tunnel: w1549 -> [w1557]
                frame #0 {
                  n459 = call "PID Distance.vi"("Distance"=90.0, "Angle"=0.0, "RightEncoder"=w1550, "LeftEncoder"=w1551, "GyroDevRef"=w1553, "RobotDriveDevRef"=w1554) -> ("RobotDriveDevRef 2"=w1552:T1)  [unwired: 2 in, 3 out]
                }
                frame #1 {
                  w1558 = 0.0
                  n460 = call <vilib>:"WPI_RobotDriveTankDrive.vi"("Right axis value"=w1558, "Left axis value"=w1558, "RobotDriveDevRef"=w1557) -> ()  [unwired: 6 in, 3 out]
                }
              }
            }
          }
        }
      }
    }
    frame "Left Scale 1" {
      n461 = flat-sequence {
        tunnel: w1564 -> [w1594]
        tunnel: w1562 -> [w1592]
        tunnel: w1563 -> [w1591]
        tunnel: w1565 -> [w1590]
        tunnel: [w1589] -> w1569
        tunnel: [w1588] -> w1568
        tunnel: [w1587] -> w1567
        tunnel: [w1586] -> w1566
        tunnel: w1561 -> [w1579]
        tunnel: w1560 -> [w1596]
        tunnel: w1569 -> [w1600]
        tunnel: w1568 -> [w1599]
        tunnel: w1567 -> [w1598]
        tunnel: w1566 -> [w1597]
        tunnel: w1559 -> [w1595]
        frame #0 {
          w1593 = 0.0 ("Left axis value")
          n462 = global read "Robot Global Data.vi" "Axes"() -> (w1572:dbl[])
          n463 = Multiply(x=w1579, y=1000.0) -> (x*y=w1580:dbl)
          n464 = global write "Robot Global Data.vi" "Lift_Position"(0.0) -> ()
          n465 = global write "Robot Global Data.vi" "Current State"(TRUE ("Current State")) -> ()
          n466 = global write "Robot Global Data.vi" "Raise_Mast"(FALSE ("Current State")) -> ()
          n467 = Wait (ms)(milliseconds to wait=u32 100) -> ()  [unwired: 1 out]
          n468 = Array To Cluster(array=w1572) -> (cluster=w1571:T15)
          n469 = Bundle By Name(cluster=w1571, "Axes[1]"=-1.0) -> (w1574:T15)
          n470 = Greater?(x=w1580, y=11000.0) -> (0:w1582:bool)
          n471 = Equal?(x=w1580, y=0.0) -> (x = y?=w1583:bool)
          n472 = Or(x=w1582, y=w1583) -> ()  [unwired: 1 out]
          n473 = Cluster To Array(cluster=w1574) -> (array=w1573:dbl[])
          n474 = call <vilib>:"WPI_GyroReset.vi"("GyroDevRef"=w1590) -> ("GyroDevRef"=w1586:T8)  [unwired: 9 in, 1 out]
          n475 = call <vilib>:"WPI_EncoderReset.vi"("EncoderDevRef"=w1592) -> ("EncoderDevRef"=w1588:T11)  [unwired: 9 in, 1 out]
          n476 = global write "Robot Global Data.vi" "Axes"(w1573) -> ()
          n477 = call <vilib>:"WPI_EncoderReset.vi"("EncoderDevRef"=w1591) -> ("EncoderDevRef"=w1587:T11)  [unwired: 9 in, 1 out]
          n478 = call <vilib>:"WPI_RobotDriveTankDrive.vi"("Right axis value"=w1593, "Left axis value"=w1593, "RobotDriveDevRef"=w1594) -> ("RobotDriveDevRef"=w1589:T1)  [unwired: 6 in, 2 out]
        }
        frame #1 {
          n479 = case shown="\"L\"" w1596 {
            tunnel: w1600 -> [w1621 w1793 w1932]
            tunnel: w1599 -> [w1618 w1790 w1934]
            tunnel: w1598 -> [w1619 w1791 w1933]
            tunnel: w1597 -> [w1620 w1792 w1931]
            tunnel: w1595 -> [w1617 _ _]
            frame "R" {
              n480 = flat-sequence {
                tunnel: w1618 -> [w1667]
                tunnel: w1619 -> [w1668]
                tunnel: w1620 -> [w1669]
                tunnel: w1621 -> [w1670]
                tunnel: [w1663] -> w1661
                tunnel: [w1664] -> w1660
                tunnel: [w1665] -> w1659
                tunnel: [w1666] -> w1658
                tunnel: [w1680] -> w1657
                tunnel: [w1679] -> w1656
                tunnel: [w1677] -> w1655
                tunnel: [w1678] -> w1654
                tunnel: w1661 -> [w1676]
                tunnel: w1660 -> [w1675]
                tunnel: w1659 -> [w1674]
                tunnel: w1658 -> [w1673]
                tunnel: w1657 -> [w1686]
                tunnel: w1656 -> [w1687]
                tunnel: [w1690] -> w1653
                tunnel: w1655 -> [w1690]
                tunnel: [w1689] -> w1652
                tunnel: w1654 -> [w1689]
                tunnel: [w1684] -> w1651
                tunnel: [w1685] -> w1650
                tunnel: w1653 -> [w1697]
                tunnel: w1652 -> [w1696]
                tunnel: [w1695] -> w1649
                tunnel: [w1694] -> w1648
                tunnel: [w1693] -> w1647
                tunnel: w1651 -> [w1693]
                tunnel: [w1691] -> w1646
                tunnel: w1650 -> [w1691]
                tunnel: w1649 -> [w1702]
                tunnel: w1648 -> [w1703]
                tunnel: w1647 -> [w1704]
                tunnel: [w1700] -> w1645
                tunnel: [w1701] -> w1644
                tunnel: w1646 -> [w1705]
                tunnel: [w1698] -> w1643
                tunnel: [w1699] -> w1642
                tunnel: w1645 -> [w1717]
                tunnel: w1644 -> [w1716]
                tunnel: [w1715] -> w1641
                tunnel: [w1714] -> w1640
                tunnel: [w1720] -> w1639
                tunnel: w1643 -> [w1720]
                tunnel: [w1719] -> w1638
                tunnel: w1642 -> [w1719]
                tunnel: w1641 -> [w1726]
                tunnel: [w1726] -> w1637
                tunnel: [w1725] -> w1636
                tunnel: [w1724] -> w1635
                tunnel: [w1723] -> w1634
                tunnel: w1640 -> [w1723]
                tunnel: w1639 -> [w1722]
                tunnel: w1638 -> [w1721]
                tunnel: w1637 -> [w1734]
                tunnel: [w1731] -> w1616
                tunnel: w1636 -> [w1733]
                tunnel: w1635 -> [w1732]
                tunnel: w1634 -> [w1735]
                tunnel: [w1730] -> w1614
                tunnel: [w1729] -> w1612
                tunnel: [w1728] -> w1610
                tunnel: w1616 -> [w1742]
                tunnel: [w1741] -> w1615
                tunnel: w1614 -> [w1739]
                tunnel: [w1738] -> w1613
                tunnel: w1612 -> [w1744]
                tunnel: [w1744] -> w1611
                tunnel: w1610 -> [w1743]
                tunnel: [w1743] -> w1609
                tunnel: w1615 -> [w1755]
                tunnel: [w1749] -> w1633
                tunnel: [w1748] -> w1632
                tunnel: w1613 -> [w1748]
                tunnel: [w1747] -> w1631
                tunnel: w1611 -> [w1747]
                tunnel: [w1746] -> w1630
                tunnel: w1609 -> [w1746]
                tunnel: w1633 -> [w1762]
                tunnel: [w1762] -> w1608
                tunnel: w1632 -> [w1761]
                tunnel: [w1761] -> w1606
                tunnel: w1631 -> [w1760]
                tunnel: [w1760] -> w1604
                tunnel: w1630 -> [w1759]
                tunnel: [w1759] -> w1602
                tunnel: w1608 -> [w1766]
                tunnel: [w1764] -> w1607
                tunnel: w1606 -> [w1765]
                tunnel: [w1763] -> w1605
                tunnel: w1604 -> [w1769]
                tunnel: [w1769] -> w1603
                tunnel: w1602 -> [w1768]
                tunnel: [w1768] -> w1601
                tunnel: w1607 -> [w1782]
                tunnel: w1605 -> [w1781]
                tunnel: w1603 -> [w1780]
                tunnel: w1601 -> [w1779]
                tunnel: [w1773] -> w1629
                tunnel: [w1772] -> w1628
                tunnel: [w1771] -> w1627
                tunnel: [w1770] -> w1626
                tunnel: w1629 -> [w1789]
                tunnel: [w1789] -> w1625
                tunnel: w1628 -> [w1788]
                tunnel: [w1788] -> w1624
                tunnel: w1627 -> [w1787]
                tunnel: [w1787] -> w1623
                tunnel: w1626 -> [w1786]
                tunnel: [w1786] -> w1622
                tunnel: w1625 -> [_]
                tunnel: w1624 -> [_]
                tunnel: w1623 -> [_]
                tunnel: w1622 -> [_]
                tunnel: w1617 -> [_]
                frame #0 {
                  n481 = global write "Robot Global Data.vi" "Raise_Mast"(FALSE ("Current State")) -> ()
                  n482 = call "PID Distance.vi"("Distance"=20.0, "Angle"=0.0, "RightEncoder"=w1667, "LeftEncoder"=w1668, "GyroDevRef"=w1669, "RobotDriveDevRef"=w1670) -> ("RightEncoder 2"=w1666:T11, "LeftEncoder 2"=w1665:T11, "GyroDevRef 2"=w1664:T8, "RobotDriveDevRef 2"=w1663:T1)  [unwired: 2 in]
                }
                frame #1 {
                  n483 = global write "Robot Global Data.vi" "Raise_Mast"(TRUE ("Current State")) -> ()
                  n484 = call "PID Distance.vi"("Distance"=225.0, "Angle"=0.0, "RightEncoder"=w1673, "LeftEncoder"=w1674, "GyroDevRef"=w1675, "RobotDriveDevRef"=w1676) -> ("RightEncoder 2"=w1677:T11, "LeftEncoder 2"=w1678:T11, "GyroDevRef 2"=w1679:T8, "RobotDriveDevRef 2"=w1680:T1)  [unwired: 2 in]
                }
                frame #2 {
                  n485 = call "PID turning.vi"("Angle"=90.0, "GyroDevRef"=w1687, "RobotDriveDevRef"=w1686) -> ("GyroDevRef 2"=w1684:T8, "RobotDriveDevRef 2"=w1685:T1)  [unwired: 7 in]
                }
                frame #3 {
                  n486 = call <vilib>:"WPI_EncoderReset.vi"("EncoderDevRef"=w1696) -> ("EncoderDevRef"=w1694:T11)  [unwired: 9 in, 1 out]
                  n487 = Wait (ms)(milliseconds to wait=u32 10) -> ()  [unwired: 1 out]
                  n488 = call <vilib>:"WPI_EncoderReset.vi"("EncoderDevRef"=w1697) -> ("EncoderDevRef"=w1695:T11)  [unwired: 9 in, 1 out]
                }
                frame #4 {
                  n489 = global read "Robot Global Data.vi" "Axes"() -> (w1709:dbl[])
                  n490 = global write "Robot Global Data.vi" "Lift_Position"(2.0) -> ()
                  n491 = call "PID Distance.vi"("Distance"=199.0, "Angle"=90.0, "RightEncoder"=w1702, "LeftEncoder"=w1703, "GyroDevRef"=w1704, "RobotDriveDevRef"=w1705) -> ("RightEncoder 2"=w1699:T11, "LeftEncoder 2"=w1698:T11, "GyroDevRef 2"=w1701:T8, "RobotDriveDevRef 2"=w1700:T1)  [unwired: 2 in]
                  n492 = Array To Cluster(array=w1709) -> (cluster=w1708:T15)
                  n493 = Bundle By Name(cluster=w1708, "Axes[1]"=-1.0) -> (w1707:T15)
                  n494 = Cluster To Array(cluster=w1707) -> (array=w1706:dbl[])
                  n495 = global write "Robot Global Data.vi" "Axes"(w1706) -> ()
                }
                frame #5 {
                  n496 = call "PID turning.vi"("Angle"=0.0, "GyroDevRef"=w1716, "RobotDriveDevRef"=w1717) -> ("GyroDevRef 2"=w1714:T8, "RobotDriveDevRef 2"=w1715:T1)  [unwired: 7 in]
                }
                frame #6 {
                  n497 = call <vilib>:"WPI_EncoderReset.vi"("EncoderDevRef"=w1722) -> ("EncoderDevRef"=w1725:T11)  [unwired: 9 in, 1 out]
                  n498 = call <vilib>:"WPI_EncoderReset.vi"("EncoderDevRef"=w1721) -> ("EncoderDevRef"=w1724:T11)  [unwired: 9 in, 1 out]
                }
                frame #7 {
                  n499 = call "PID Distance.vi"("Distance"=38.0, "Angle"=0.0, "RightEncoder"=w1732, "LeftEncoder"=w1733, "GyroDevRef"=w1735, "RobotDriveDevRef"=w1734) -> ("RightEncoder 2"=w1728:T11, "LeftEncoder 2"=w1729:T11, "GyroDevRef 2"=w1730:T8, "RobotDriveDevRef 2"=w1731:T1)  [unwired: 2 in]
                  n500 = global write "Robot Global Data.vi" "Lift_Position"(3.0) -> ()
                }
                frame #8 {
                  n501 = call "PID turning.vi"("Angle"=-20.0, "GyroDevRef"=w1739, "RobotDriveDevRef"=w1742) -> ("GyroDevRef 2"=w1738:T8, "RobotDriveDevRef 2"=w1741:T1)  [unwired: 7 in]
                }
                frame #9 {
                  w1756 = 0.0 ("Left axis value")
                  n502 = global read "Robot Global Data.vi" "Axes"() -> (w1751:dbl[])
                  n503 = Wait (ms)(milliseconds to wait=u32 300) -> ()  [unwired: 1 out]
                  n504 = Array To Cluster(array=w1751) -> (cluster=w1750:T15)
                  n505 = Bundle By Name(cluster=w1750, "Axes[1]"=0.25) -> (w1753:T15)
                  n506 = Cluster To Array(cluster=w1753) -> (array=w1752:dbl[])
                  n507 = call <vilib>:"WPI_RobotDriveTankDrive.vi"("Right axis value"=w1756, "Left axis value"=w1756, "RobotDriveDevRef"=w1755) -> ("RobotDriveDevRef"=w1749:T1)  [unwired: 6 in, 2 out]
                  n508 = global write "Robot Global Data.vi" "Axes"(w1752) -> ()
                }
                frame #10 {
                  n509 = global write "Robot Global Data.vi" "Current State"(FALSE ("Current State")) -> ()
                  n510 = Wait (ms)(milliseconds to wait=u32 400) -> ()  [unwired: 1 out]
                }
                frame #11 {
                  n511 = call "PID turning.vi"("Angle"=0.0, "GyroDevRef"=w1765, "RobotDriveDevRef"=w1766) -> ("GyroDevRef 2"=w1763:T8, "RobotDriveDevRef 2"=w1764:T1)  [unwired: 7 in]
                }
                frame #12 {
                  n512 = global read "Robot Global Data.vi" "Axes"() -> (w1778:dbl[])
                  n513 = call "PID Distance.vi"("Distance"=20.0, "Angle"=0.0, "RightEncoder"=w1779, "LeftEncoder"=w1780, "GyroDevRef"=w1781, "RobotDriveDevRef"=w1782) -> ("RightEncoder 2"=w1770:T11, "LeftEncoder 2"=w1771:T11, "GyroDevRef 2"=w1772:T8, "RobotDriveDevRef 2"=w1773:T1)  [unwired: 2 in]
                  n514 = Array To Cluster(array=w1778) -> (cluster=w1777:T15)
                  n515 = Bundle By Name(cluster=w1777, "Axes[1]"=-1.0) -> (w1776:T15)
                  n516 = Cluster To Array(cluster=w1776) -> (array=w1775:dbl[])
                  n517 = global write "Robot Global Data.vi" "Axes"(w1775) -> ()
                }
                frame #13 {
                  n518 = global write "Robot Global Data.vi" "Lift_Position"(1.0) -> ()
                }
                frame #14 {
                }
              }
            }
            frame "L" {
              n519 = flat-sequence {
                tunnel: [w1841] -> w1833
                tunnel: [w1838] -> w1832
                tunnel: [w1839] -> w1831
                tunnel: [w1840] -> w1830
                tunnel: w1793 -> [w1837]
                tunnel: w1792 -> [w1836]
                tunnel: w1791 -> [w1835]
                tunnel: w1790 -> [w1834]
                tunnel: [w1848] -> w1829
                tunnel: [w1845] -> w1828
                tunnel: [w1846] -> w1827
                tunnel: [w1847] -> w1826
                tunnel: w1833 -> [w1852]
                tunnel: w1832 -> [w1849]
                tunnel: w1831 -> [w1850]
                tunnel: w1830 -> [w1851]
                tunnel: [w1859] -> w1822
                tunnel: [w1858] -> w1823
                tunnel: [w1856] -> w1824
                tunnel: [w1857] -> w1825
                tunnel: w1829 -> [w1863]
                tunnel: w1828 -> [w1860]
                tunnel: w1827 -> [w1861]
                tunnel: w1826 -> [w1862]
                tunnel: [w1871] -> w1821
                tunnel: w1825 -> [w1867]
                tunnel: w1824 -> [w1868]
                tunnel: w1823 -> [w1870]
                tunnel: w1822 -> [w1872]
                tunnel: [w1869] -> w1820
                tunnel: [w1868] -> w1819
                tunnel: [w1867] -> w1818
                tunnel: w1821 -> [w1882]
                tunnel: [w1882] -> w1817
                tunnel: w1820 -> [w1881]
                tunnel: [w1881] -> w1816
                tunnel: [w1880] -> w1815
                tunnel: [w1879] -> w1814
                tunnel: w1819 -> [w1877]
                tunnel: w1818 -> [w1876]
                tunnel: w1817 -> [w1888]
                tunnel: [w1886] -> w1813
                tunnel: w1816 -> [w1887]
                tunnel: [w1885] -> w1812
                tunnel: w1815 -> [w1890]
                tunnel: w1814 -> [w1889]
                tunnel: [w1884] -> w1811
                tunnel: [w1883] -> w1810
                tunnel: w1813 -> [w1897]
                tunnel: [w1896] -> w1809
                tunnel: [w1895] -> w1808
                tunnel: w1812 -> [w1895]
                tunnel: [w1894] -> w1807
                tunnel: w1811 -> [w1894]
                tunnel: [w1893] -> w1806
                tunnel: w1810 -> [w1893]
                tunnel: [w1908] -> w1805
                tunnel: w1809 -> [w1908]
                tunnel: [w1907] -> w1804
                tunnel: w1808 -> [w1907]
                tunnel: [w1906] -> w1803
                tunnel: w1807 -> [w1906]
                tunnel: [w1905] -> w1802
                tunnel: w1806 -> [w1905]
                tunnel: w1805 -> [w1913]
                tunnel: w1804 -> [w1914]
                tunnel: [w1914] -> w1801
                tunnel: [w1913] -> w1800
                tunnel: [w1912] -> w1799
                tunnel: w1803 -> [w1912]
                tunnel: [w1911] -> w1798
                tunnel: w1802 -> [w1911]
                tunnel: [w1927] -> w1797
                tunnel: w1801 -> [w1929]
                tunnel: w1800 -> [w1928]
                tunnel: w1799 -> [w1924]
                tunnel: w1798 -> [w1923]
                tunnel: [w1922] -> w1796
                tunnel: [w1921] -> w1795
                tunnel: [w1920] -> w1794
                tunnel: w1794 -> [_]
                tunnel: w1795 -> [_]
                tunnel: w1796 -> [_]
                tunnel: w1797 -> [_]
                frame #0 {
                  n520 = call "PID Distance.vi"("Distance"=20.0, "Angle"=-2.0, "RightEncoder"=w1834, "LeftEncoder"=w1835, "GyroDevRef"=w1836, "RobotDriveDevRef"=w1837) -> ("RightEncoder 2"=w1838:T11, "LeftEncoder 2"=w1839:T11, "GyroDevRef 2"=w1840:T8, "RobotDriveDevRef 2"=w1841:T1)  [unwired: 2 in]
                }
                frame #1 {
                  n521 = call "PID Distance.vi"("Distance"=100.0, "Angle"=-2.0, "RightEncoder"=w1849, "LeftEncoder"=w1850, "GyroDevRef"=w1851, "RobotDriveDevRef"=w1852) -> ("RightEncoder 2"=w1845:T11, "LeftEncoder 2"=w1846:T11, "GyroDevRef 2"=w1847:T8, "RobotDriveDevRef 2"=w1848:T1)  [unwired: 2 in]
                  n522 = global write "Robot Global Data.vi" "Raise_Mast"(TRUE ("Current State")) -> ()
                }
                frame #2 {
                  n523 = global write "Robot Global Data.vi" "Lift_Position"(2.0) -> ()
                  n524 = call "PID Distance.vi"("Distance"=300.0, "Angle"=-2.0, "RightEncoder"=w1860, "LeftEncoder"=w1861, "GyroDevRef"=w1862, "RobotDriveDevRef"=w1863) -> ("RightEncoder 2"=w1856:T11, "LeftEncoder 2"=w1857:T11, "GyroDevRef 2"=w1858:T8, "RobotDriveDevRef 2"=w1859:T1)  [unwired: 2 in]
                  n525 = global write "Robot Global Data.vi" "Raise_Mast"(TRUE ("Current State")) -> ()
                }
                frame #3 {
                  n526 = call "PID turning.vi"("Angle"=90.0, "GyroDevRef"=w1870, "RobotDriveDevRef"=w1872) -> ("GyroDevRef 2"=w1869:T8, "RobotDriveDevRef 2"=w1871:T1)  [unwired: 7 in]
                  n527 = global write "Robot Global Data.vi" "Lift_Position"(3.0) -> ()
                  n528 = global write "Robot Global Data.vi" "Raise_Mast"(TRUE ("Current State")) -> ()
                }
                frame #4 {
                  n529 = call <vilib>:"WPI_EncoderReset.vi"("EncoderDevRef"=w1876) -> ("EncoderDevRef"=w1879:T11)  [unwired: 9 in, 1 out]
                  n530 = Wait (ms)(milliseconds to wait=u32 100) -> ()  [unwired: 1 out]
                  n531 = call <vilib>:"WPI_EncoderReset.vi"("EncoderDevRef"=w1877) -> ("EncoderDevRef"=w1880:T11)  [unwired: 9 in, 1 out]
                }
                frame #5 {
                  n532 = call "PID Distance.vi"("Distance"=25.0, "Angle"=90.0, "RightEncoder"=w1890, "LeftEncoder"=w1889, "GyroDevRef"=w1887, "RobotDriveDevRef"=w1888) -> ("RightEncoder 2"=w1883:T11, "LeftEncoder 2"=w1884:T11, "GyroDevRef 2"=w1885:T8, "RobotDriveDevRef 2"=w1886:T1)  [unwired: 2 in]
                }
                frame #6 {
                  w1898 = 0.0 ("Left axis value")
                  n533 = global read "Robot Global Data.vi" "Axes"() -> (w1901:dbl[])
                  n534 = Wait (ms)(milliseconds to wait=u32 500) -> ()  [unwired: 1 out]
                  n535 = Array To Cluster(array=w1901) -> (cluster=w1900:T15)
                  n536 = Bundle By Name(cluster=w1900, "Axes[1]"=0.25) -> (w1903:T15)
                  n537 = Cluster To Array(cluster=w1903) -> (array=w1902:dbl[])
                  n538 = call <vilib>:"WPI_RobotDriveTankDrive.vi"("Right axis value"=w1898, "Left axis value"=w1898, "RobotDriveDevRef"=w1897) -> ("RobotDriveDevRef"=w1896:T1)  [unwired: 6 in, 2 out]
                  n539 = global write "Robot Global Data.vi" "Axes"(w1902) -> ()
                }
                frame #7 {
                  n540 = global write "Robot Global Data.vi" "Current State"(FALSE ("Current State")) -> ()
                  n541 = Wait (ms)(milliseconds to wait=u32 400) -> ()  [unwired: 1 out]
                }
                frame #8 {
                  n542 = global read "Robot Global Data.vi" "Axes"() -> (w1916:dbl[])
                  n543 = Array To Cluster(array=w1916) -> (cluster=w1915:T15)
                  n544 = Bundle By Name(cluster=w1915, "Axes[1]"=-1.0) -> (w1918:T15)
                  n545 = Cluster To Array(cluster=w1918) -> (array=w1917:dbl[])
                  n546 = global write "Robot Global Data.vi" "Axes"(w1917) -> ()
                }
                frame #9 {
                  n547 = call "PID Distance.vi"("Distance"=0.0, "Angle"=90.0, "RightEncoder"=w1923, "LeftEncoder"=w1924, "GyroDevRef"=w1929, "RobotDriveDevRef"=w1928) -> ("RightEncoder 2"=w1920:T11, "LeftEncoder 2"=w1921:T11, "GyroDevRef 2"=w1922:T8, "RobotDriveDevRef 2"=w1927:T1)  [unwired: 2 in]
                }
                frame #10 {
                  n548 = global write "Robot Global Data.vi" "Lift_Position"(1.0) -> ()
                }
              }
            }
            frame Default {
              n549 = flat-sequence {
                tunnel: w1932 -> [w1940]
                tunnel: w1931 -> [w1939]
                tunnel: w1933 -> [w1937]
                tunnel: [w1938] -> w1935
                tunnel: w1934 -> [w1936]
                tunnel: w1935 -> [w1943]
                frame #0 {
                  n550 = call "PID Distance.vi"("Distance"=90.0, "Angle"=0.0, "RightEncoder"=w1936, "LeftEncoder"=w1937, "GyroDevRef"=w1939, "RobotDriveDevRef"=w1940) -> ("RobotDriveDevRef 2"=w1938:T1)  [unwired: 2 in, 3 out]
                }
                frame #1 {
                  w1944 = 0.0
                  n551 = call <vilib>:"WPI_RobotDriveTankDrive.vi"("Right axis value"=w1944, "Left axis value"=w1944, "RobotDriveDevRef"=w1943) -> ()  [unwired: 6 in, 3 out]
                }
              }
            }
          }
        }
      }
    }
    frame "Left Scale 2" {
      n552 = flat-sequence {
        tunnel: w1946 -> [w1980]
        tunnel: w1949 -> [w1978]
        tunnel: w1948 -> [w1977]
        tunnel: w1947 -> [w1976]
        tunnel: [w1975] -> w1955
        tunnel: [w1974] -> w1954
        tunnel: [w1973] -> w1953
        tunnel: [w1972] -> w1952
        tunnel: w1945 -> [w1965]
        tunnel: w1950 -> [w1982]
        tunnel: w1955 -> [w1986]
        tunnel: w1954 -> [w1985]
        tunnel: w1953 -> [w1984]
        tunnel: w1952 -> [w1983]
        tunnel: w1951 -> [w1981]
        frame #0 {
          w1979 = 0.0 ("Left axis value")
          n553 = global read "Robot Global Data.vi" "Axes"() -> (w1958:dbl[])
          n554 = Multiply(x=w1965, y=1000.0) -> (x*y=w1966:dbl)
          n555 = global write "Robot Global Data.vi" "Lift_Position"(0.0) -> ()
          n556 = global write "Robot Global Data.vi" "Raise_Mast"(FALSE ("Current State")) -> ()
          n557 = global write "Robot Global Data.vi" "Current State"(TRUE ("Current State")) -> ()
          n558 = Wait (ms)(milliseconds to wait=u32 100) -> ()  [unwired: 1 out]
          n559 = Array To Cluster(array=w1958) -> (cluster=w1957:T15)
          n560 = Bundle By Name(cluster=w1957, "Axes[1]"=-1.0) -> (w1960:T15)
          n561 = Greater?(x=w1966, y=11000.0) -> (0:w1968:bool)
          n562 = Equal?(x=w1966, y=0.0) -> (x = y?=w1969:bool)
          n563 = Or(x=w1968, y=w1969) -> ()  [unwired: 1 out]
          n564 = Cluster To Array(cluster=w1960) -> (array=w1959:dbl[])
          n565 = call <vilib>:"WPI_GyroReset.vi"("GyroDevRef"=w1976) -> ("GyroDevRef"=w1972:T8)  [unwired: 9 in, 1 out]
          n566 = call <vilib>:"WPI_EncoderReset.vi"("EncoderDevRef"=w1978) -> ("EncoderDevRef"=w1974:T11)  [unwired: 9 in, 1 out]
          n567 = global write "Robot Global Data.vi" "Axes"(w1959) -> ()
          n568 = call <vilib>:"WPI_EncoderReset.vi"("EncoderDevRef"=w1977) -> ("EncoderDevRef"=w1973:T11)  [unwired: 9 in, 1 out]
          n569 = call <vilib>:"WPI_RobotDriveTankDrive.vi"("Right axis value"=w1979, "Left axis value"=w1979, "RobotDriveDevRef"=w1980) -> ("RobotDriveDevRef"=w1975:T1)  [unwired: 6 in, 2 out]
        }
        frame #1 {
          n570 = case shown="\"R\"" w1982 {
            tunnel: w1986 -> [w1988 w2334 w2661]
            tunnel: w1985 -> [w1991 w2331 w2663]
            tunnel: w1984 -> [w1990 w2332 w2662]
            tunnel: w1983 -> [w1989 w2333 w2660]
            tunnel: w1981 -> [w1987 w2330 _]
            frame "R" {
              n571 = flat-sequence {
                tunnel: w1991 -> [w2053]
                tunnel: w1990 -> [w2054]
                tunnel: w1989 -> [w2055]
                tunnel: w1988 -> [w2056]
                tunnel: [w2049] -> w2047
                tunnel: [w2050] -> w2046
                tunnel: [w2051] -> w2045
                tunnel: [w2052] -> w2044
                tunnel: [w2066] -> w2043
                tunnel: [w2065] -> w2042
                tunnel: [w2063] -> w2041
                tunnel: [w2064] -> w2040
                tunnel: w2047 -> [w2062]
                tunnel: w2046 -> [w2061]
                tunnel: w2045 -> [w2060]
                tunnel: w2044 -> [w2059]
                tunnel: w2043 -> [w2072]
                tunnel: w2042 -> [w2073]
                tunnel: [w2076] -> w2039
                tunnel: w2041 -> [w2076]
                tunnel: [w2075] -> w2038
                tunnel: w2040 -> [w2075]
                tunnel: [w2070] -> w2037
                tunnel: [w2071] -> w2036
                tunnel: w2039 -> [w2083]
                tunnel: w2038 -> [w2082]
                tunnel: [w2081] -> w2035
                tunnel: [w2080] -> w2034
                tunnel: [w2079] -> w2033
                tunnel: w2037 -> [w2079]
                tunnel: [w2077] -> w2032
                tunnel: w2036 -> [w2077]
                tunnel: w2035 -> [w2088]
                tunnel: w2034 -> [w2089]
                tunnel: w2033 -> [w2090]
                tunnel: [w2086] -> w2031
                tunnel: [w2087] -> w2030
                tunnel: w2032 -> [w2091]
                tunnel: [w2084] -> w2029
                tunnel: [w2085] -> w2028
                tunnel: w2031 -> [w2103]
                tunnel: w2030 -> [w2102]
                tunnel: [w2101] -> w2027
                tunnel: [w2100] -> w2026
                tunnel: [w2106] -> w2025
                tunnel: w2029 -> [w2106]
                tunnel: [w2105] -> w2024
                tunnel: w2028 -> [w2105]
                tunnel: w2027 -> [w2112]
                tunnel: [w2112] -> w2023
                tunnel: [w2111] -> w2022
                tunnel: [w2110] -> w2021
                tunnel: [w2109] -> w2020
                tunnel: w2026 -> [w2109]
                tunnel: w2025 -> [w2108]
                tunnel: w2024 -> [w2107]
                tunnel: w2023 -> [w2120]
                tunnel: [w2117] -> w2019
                tunnel: w2022 -> [w2119]
                tunnel: w2021 -> [w2118]
                tunnel: w2020 -> [w2121]
                tunnel: [w2116] -> w2018
                tunnel: [w2115] -> w2017
                tunnel: [w2114] -> w2016
                tunnel: w2019 -> [w2128]
                tunnel: [w2127] -> w2015
                tunnel: w2018 -> [w2125]
                tunnel: [w2124] -> w2014
                tunnel: w2017 -> [w2130]
                tunnel: [w2130] -> w2013
                tunnel: w2016 -> [w2129]
                tunnel: [w2129] -> w2012
                tunnel: w2015 -> [w2141]
                tunnel: [w2135] -> w2011
                tunnel: [w2134] -> w2010
                tunnel: w2014 -> [w2134]
                tunnel: [w2133] -> w2009
                tunnel: w2013 -> [w2133]
                tunnel: [w2132] -> w2008
                tunnel: w2012 -> [w2132]
                tunnel: w2011 -> [w2148]
                tunnel: [w2148] -> w2007
                tunnel: w2010 -> [w2147]
                tunnel: [w2147] -> w2006
                tunnel: w2009 -> [w2146]
                tunnel: [w2146] -> w2005
                tunnel: w2008 -> [w2145]
                tunnel: [w2145] -> w2004
                tunnel: w2007 -> [w2152]
